vi "Load Additional Function.vi"(8 "error in (no error)":errorcluster, 10 "Array of Function Paths":path[](array[path]), 11 "Controller in":refnum<class "Controller.lvclass">) -> (0 "error out":errorcluster, 3 "Controller out":refnum<class "Controller.lvclass">)   [LabVIEW 2016, in "Controller Actor.lvlib" / "Controller.lvclass"]
uses:
  <userlib>/Common Components/Controller/Controller.lvclass
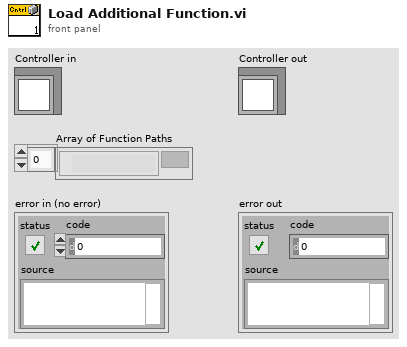
[diagram p1: front panel]
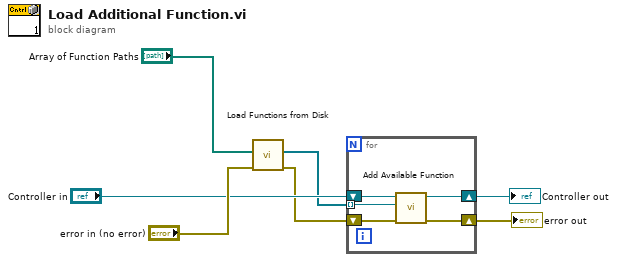
[diagram p0: block diagram]
diagram:
  n1 = call <userlib>:"Load Functions from Disk.vi"("error in (no error)"="error in (no error)", "Array of paths (folders to scan or explicit files)"="Array of Function Paths") -> ("error out"=w2:errorcluster, "Available Functions"=w1:refnum<class "Function.lvclass">[])  [unwired: 8 in]
  n2 = for {
    tunnel: w1 -> [w10] mode=indexing
    shift-right: [w11] -> w6
    shift-left: "Controller in" -> [w12]
    shift-right: [w8] -> w7
    shift-left: w2 -> [w9]
    n3 = call <userlib>:"Add Available Function.vi"("error in (no error)"=w9, "Function.lvclass"=w10, "Controller in"=w12) -> ("error out"=w8:errorcluster, "Controller out"=w11:refnum<class "Controller.lvclass">)  [unwired: 7 in]
  }
  "error out" <- w7
  "Controller out" <- w6
